vi "Set Sensor Calibration Coeffs.vi"(9 "Select Probe":i32, 10 "CalibrCoefArray":dbl[](array[numeric])) -> ()   [LabVIEW 2015, in "Tool Cfg.lvlib"]
uses:
  Tool Cfg.lvlib
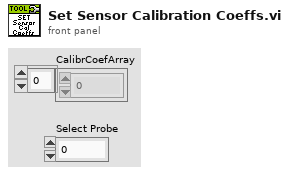
[diagram p1: front panel]
types:
  T1 = typedef "Tool Cfg.lvlib/_SensorConfigParams Cluster--typedef.ctl" = cluster{"Total Pixels":u16, "Positive  Peaks":bool, "CalibrCoefArray":dbl[], "Start Idx":u16, "End Idx":u16}
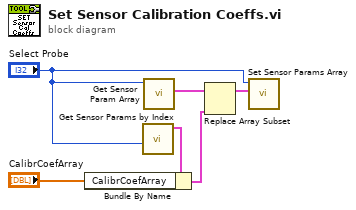
[diagram p0: block diagram]
diagram:
  n1 = call "Get Sensor Params by Index.vi"("index"="Select Probe") -> ("Sensor Cfg Params"=w2:T1)  [unwired: 10 in]
  n2 = Bundle By Name(cluster=w2, "CalibrCoefArray"="CalibrCoefArray") -> (w4:T1)
  n3 = call "Get Sensor Param Array.vi"("Select Probe"="Select Probe") -> ("Sensor Block.SensorCfgParams Array"=w5:T1[])  [unwired: 9 in, 1 out]
  n4 = Replace Array Subset(array=w5, new element=w4) -> (w3:T1[])  [unwired: 1 in]
  n5 = call "Set Sensor Params Array.vi"("SensorCfgParams Array"=w3, "Select Probe"="Select Probe") -> ()  [unwired: 10 in]
